vi "Console Entry.vi"(6 "Error In":errorcluster, 8 "Data In":T1={"Console log"="", "GUI_Events"={"To_GUI-Producer"=refnum, "To_GUI-Error_message"=refnum, "To_GUI-msg_list"=refnum, "To_GUI-Session"=refnum, "To_GUI-Pre-Session"=refnum, "To_GUI-Consumer"=refnum}, "Function_Queue"={"Queue_MIDI_Handler"=refnum, "Queue_Session"=refnum, "Queue_Producer"=refnum, "Queue_Consumer"=refnum}, "Timout-Time[ms]"=0, "MIDI-Messages"=[], "Com Session State"=enum."Active Session", "Result Data"={"Diff"=[], "Tx Byte"=[], "Rx Byte"=[], "Send Log"=[], "Parsed Data"={"Tx MIDI Tag"=[], "Tx MIDI Parsed Data"=[], "Tx Error"=[], "Tx Running States"=[], "Rx MIDI Tag"=[], "Rx MIDI Parsed Data"=[], "Rx Error"=[], "Rx Running States"=[], "Diff"=[]}}, "Get #"=[], "CPU(ms)"=0}, 11 "Console Entry":string) -> (0 "Data out":T1={"Console log"="", "GUI_Events"={"To_GUI-Producer"=refnum, "To_GUI-Error_message"=refnum, "To_GUI-msg_list"=refnum, "To_GUI-Session"=refnum, "To_GUI-Pre-Session"=refnum, "To_GUI-Consumer"=refnum}, "Function_Queue"={"Queue_MIDI_Handler"=refnum, "Queue_Session"=refnum, "Queue_Producer"=refnum, "Queue_Consumer"=refnum}, "Timout-Time[ms]"=0, "MIDI-Messages"=[], "Com Session State"=enum."Active Session", "Result Data"={"Diff"=[], "Tx Byte"=[], "Rx Byte"=[], "Send Log"=[], "Parsed Data"={"Tx MIDI Tag"=[], "Tx MIDI Parsed Data"=[], "Tx Error"=[], "Tx Running States"=[], "Rx MIDI Tag"=[], "Rx MIDI Parsed Data"=[], "Rx Error"=[], "Rx Running States"=[], "Diff"=[]}}, "Get #"=[], "CPU(ms)"=0})   [LabVIEW 2019]
doc: "Adds a new entry to a console log, if an error has occured it will also be logged."
uses:
  Controls/Application_Data.ctl
  Controls/App_Events.ctl
  Controls/App_Queues.ctl
  Controls/Application_Message.ctl
  Controls/Application_State.ctl
  MIDI/Controls/MIDI-Message_Array.ctl
  MIDI/Controls/MIDI-Message_Cluster.ctl
  MIDI/Controls/Meta_Commands.ctl
  Producer/Controls/Session_State.ctl
  Consumer/Controls/Consumer_Result.ctl
  Consumer/Controls/Parsed_Data.ctl
panel:
  out "Revision Number":u32
  out "Code Size":u32
  out "VI Path":path
  out "VI-filename":string
  out "Timestamp":string
  out "Console log in":string
  out "Console log out":string
  # "VI Input"
  # "VI Output"
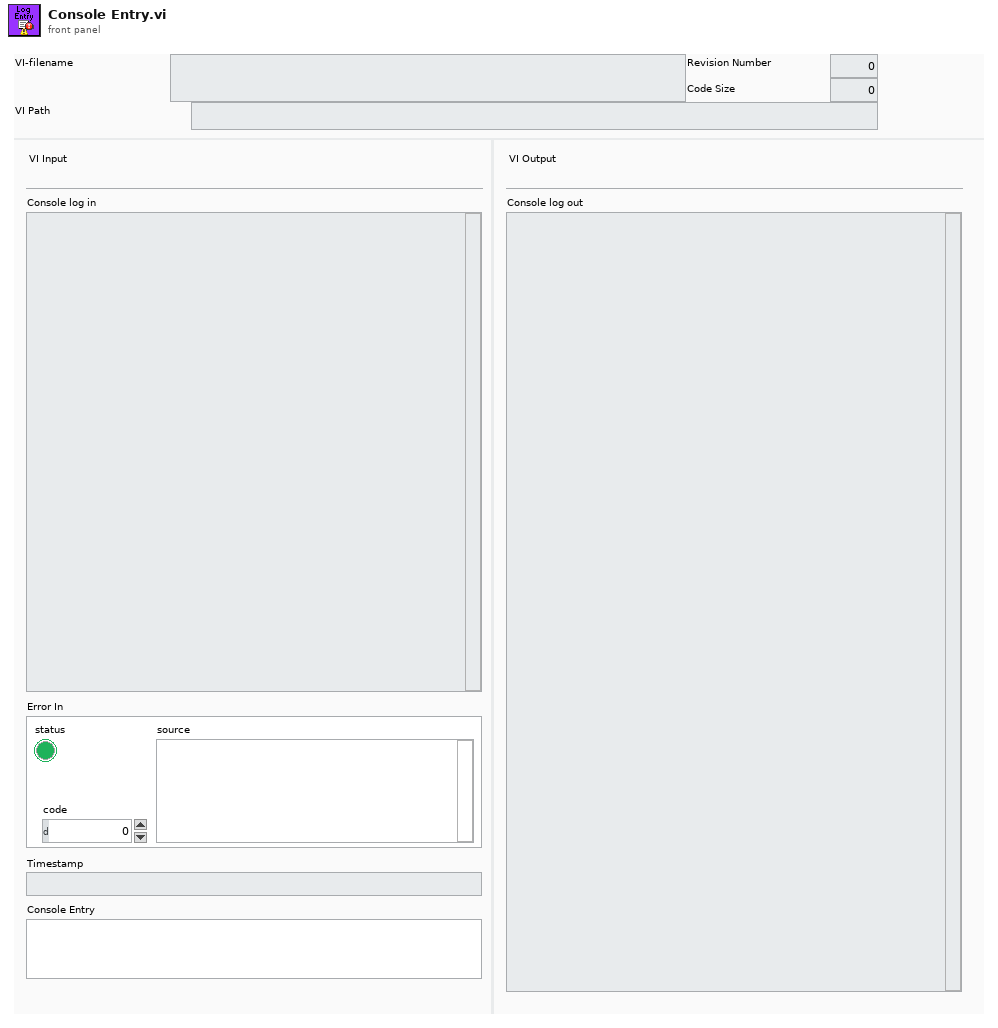
[diagram p1: front panel]
types:
  T1 = typedef "Application_Data.ctl" = cluster{"Console log":string, "GUI_Events":T2, "Function_Queue":T3, "Timout-Time[ms]":i32, "MIDI-Messages":T4, "Com Session State":T7, "Result Data":T8, "Get #":bool[], "CPU(ms)":u32}
  T2 = typedef "App_Events.ctl" = cluster{"To_GUI-Producer":refnum<user-event>, "To_GUI-Error_message":refnum<user-event>, "To_GUI-msg_list":refnum<user-event>, "To_GUI-Session":refnum<user-event>, "To_GUI-Pre-Session":refnum<user-event>, "To_GUI-Consumer":refnum<user-event>}
  T3 = typedef "App_Queues.ctl" = cluster{"Queue_MIDI_Handler":refnum<queue>, "Queue_Session":refnum<queue>, "Queue_Producer":refnum<queue>, "Queue_Consumer":refnum<queue>}
  T4 = typedef "MIDI-Message_Array.ctl" = T5[]
  T5 = typedef "MIDI-Message_Cluster.ctl" = cluster{"Message Name":string, "Meta value":i32, "Datastring":string, "Datatype":T6}
  T6 = typedef "Meta_Commands.ctl" = enum16{"No Data", "Pause", "Loop", "Wait for Rx", "Delay", "Break", "MIDI"}
  T7 = typedef "Session_State.ctl" = enum16{"Wait to begin", "Active Session", "Pause", "Wait for Response", "Stop", "Restart", "Inspect", "Exit"}
  T8 = typedef "Consumer_Result.ctl" = cluster{"Diff":bool[], "Tx Byte":string[], "Rx Byte":string[], "Send Log":string[], "Parsed Data":T9}
  T9 = typedef "Parsed_Data.ctl" = cluster{"Tx MIDI Tag":string[], "Tx MIDI Parsed Data":string[], "Tx Error":bool[], "Tx Running States":string[], "Rx MIDI Tag":string[], "Rx MIDI Parsed Data":string[], "Rx Error":bool[], "Rx Running States":string[], "Diff":bool[]}
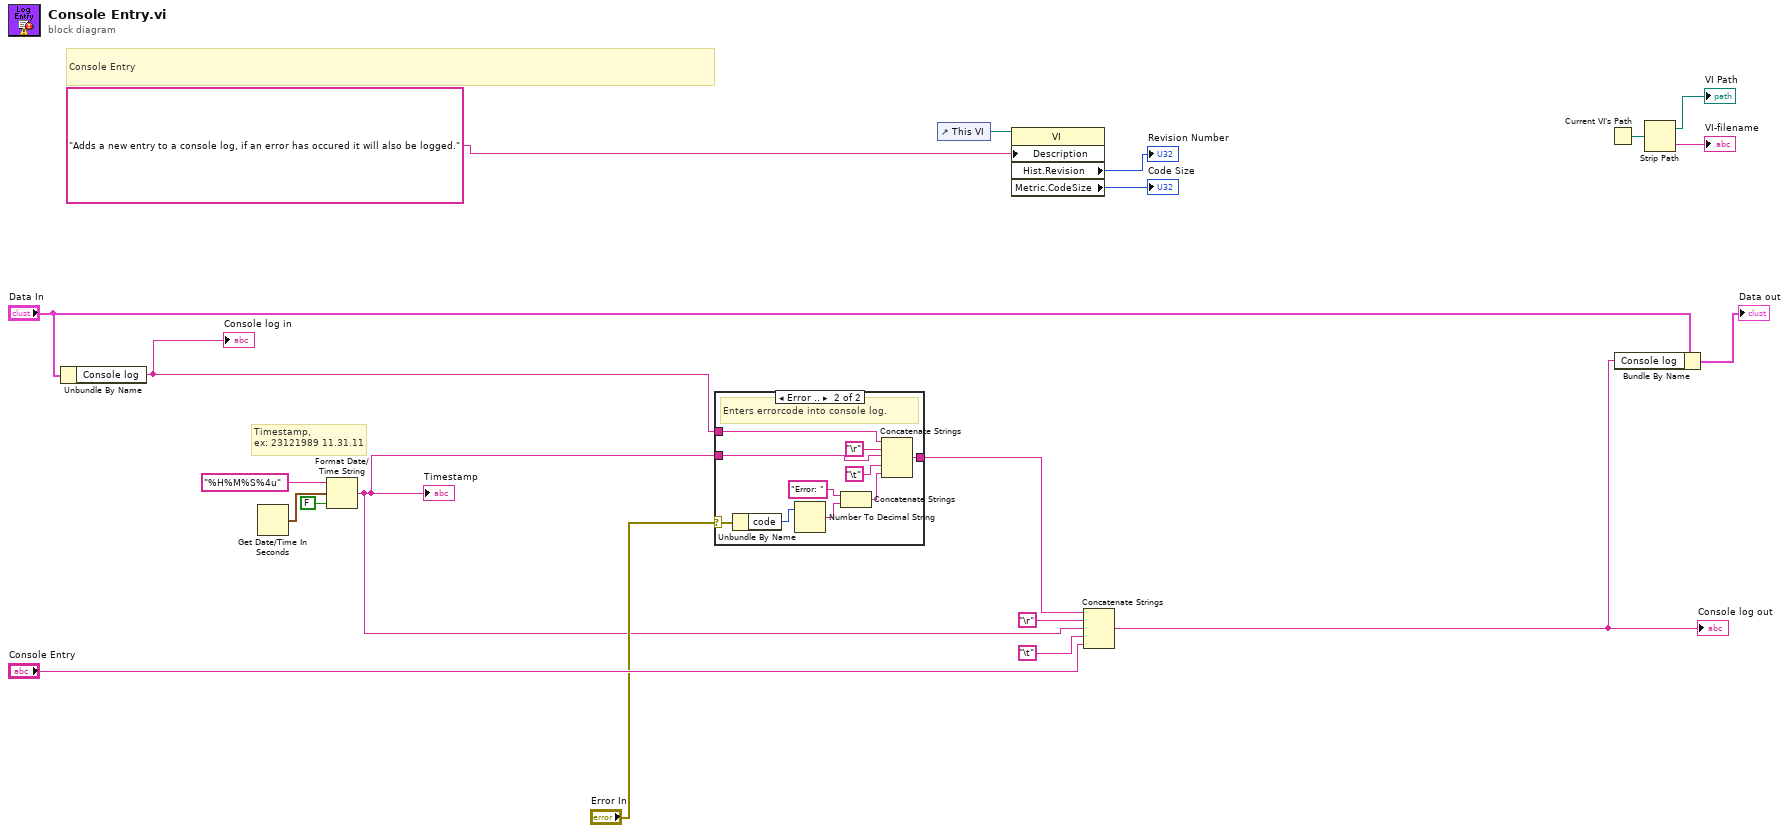
[diagram p0: block diagram]
diagram:
  # "Timestamp, \nex: 23121989 11.31.11"
  # "Console Entry"
  n1 = Unbundle By Name("Data In") -> ("Console log"=w7:string)
  "Console log in" <- w7
  n2 = Get Date/Time In Seconds() -> (seconds since 1Jan1904=w11:timestamp)
  n3 = Format Date/Time String(time format string (%c)="%H%M%S%4u", seconds (now)=w11, UTC format=FALSE) -> (date/time string=w6:string)
  "Timestamp" <- w6
  n4 = case shown="Error .." "Error In" {
    selector: "Error In" -> [_ w22]
    tunnel: w7 -> [w21 w27]
    tunnel: w6 -> [_ w25]
    tunnel: [w21 w23] -> w5
    frame No Error {
    }
    frame Error {
      # "Enters errorcode into console log."
      n5 = Unbundle By Name(w22) -> ("code"=w31:i32)
      n6 = Number To Decimal String(number=w31) -> (decimal integer string=w30:string)  [unwired: 1 in]
      n7 = Concatenate Strings("Error: " ("string"), w30) -> (w29:string)
      n8 = Concatenate Strings(w27, "\r", w25, "\t", w29) -> (w23:string)
    }
  }
  n9 = control-ref of="This VI"() -> (w2:refnum<vi>)
  n10 = property class="VI"(reference=w2, "Description"="Adds a new entry to a console log, if an error has occured it will also be logged.") -> ("Hist.Revision"=→"Revision Number":u32, "Metric.CodeSize"=→"Code Size":u32)  [unwired: 1 in, 2 out]
  n11 = Concatenate Strings(w5, "\r", w6, "\t", "Console Entry") -> (w16:string)
  "Console log out" <- w16
  n12 = Current VI's Path() -> (path=w20:path)
  n13 = Bundle By Name(cluster="Data In", "Console log"=w16) -> (→"Data out":T1)
  n14 = Strip Path(path=w20) -> (stripped path=→"VI Path":path, name=→"VI-filename":string)
